vi "DrawUserEvent.vi"(11 "PictureBox":refnum<k24>(container)) -> ()   [LabVIEW 2016]
uses:
  System.Windows.Forms
  System.Drawing
panel:
  in  "stop":bool
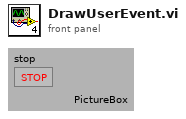
[diagram p1: front panel]
types:
  T1 = cluster{"Event Common Data":cluster{"Event Source":i32, "Event Type":u32, "Time Stamp":u32}, "Control Ref":refnum<k24>, "Event Data":cluster{"sender":refnum<k24>, "e":refnum<k24>}}
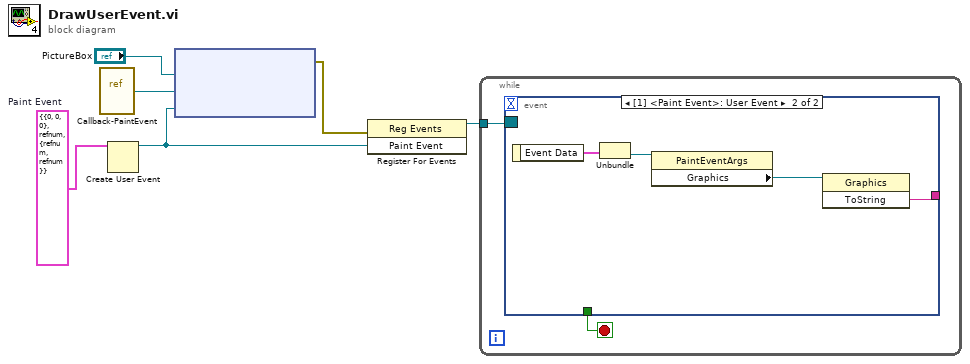
[diagram p0: block diagram]
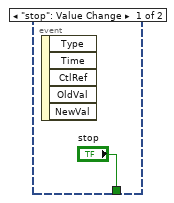
[diagram p2: hidden frame]
diagram:
  w1 = T1 {"Event Common Data"={"Event Source"=0, "Event Type"=0, "Time Stamp"=0}, "Control Ref"=refnum, "Event Data"={"sender"=refnum, "e"=refnum}}  # Paint Event
  n1 = vi-ref "Callback-PaintEvent.vi"() -> ("vi reference"=w6:refnum<vi>)
  n2 = Create User Event(user event datatype=w1) -> (user event=w5:refnum<user-event>)  [unwired: 1 in, 1 out]
  n3 = node("PictureBox", w6, w5) -> (w2:errorcluster)  [unwired: 2 in, 1 out]
  n4 = register-events(error in=w2, w5) -> (reference out=w4:refnum<event-registration>)  [unwired: 1 in, 1 out]
  n5 = while {
    tunnel: w4 -> [w8]
    stop <- w7 stop-if-true
    n6 = event shown="[1] <Paint Event>: User Event" {
      selector: w8 -> [_ _]
      dyn-events: _ -> [_ _]
      timeout: _ -> [_ _]
      tunnel: ["stop" _] -> w7
      tunnel: [_ w10] -> _
      event "stop": Value Change {
        n7 = event-data() -> ()  [unwired: 1 in, 5 out]
      }
      event User Event {
        n8 = event-data() -> ("Event Data"=w13:cluster{"sender":refnum<k24>, "e":refnum<k24>})  [unwired: 1 in]
        n9 = Unbundle(w13) -> ("e"=w12:refnum<k24>)  [unwired: 1 out]
        n10 = property class="PaintEventArgs"(reference=w12) -> ("Graphics"=w11:refnum<k24>)  [unwired: 1 in, 2 out]
        n11 = invoke class="Graphics" method="ToString"(reference=w11) -> ("ToString"=w10:string)  [unwired: 2 in, 2 out]
      }
    }
  }
